vi "MacroFileIO.vi"(0 "New Path IN":path, 1 "MacroFileIO_Command":T3, 5 "Settings File Name IN":string, 7 "Settings Data IN":T2[](array[typedef]), 9 "Setting File Type":T1=enum."Configuration Settings", 11 "Error In":errorcluster, 12 "Macro Text IN":string) -> (3 "File IO Cancelled/NotFound?":bool, 4 "Macro File Path OUT":path, 6 "Temp File path":path, 10 "List of Settings Files in Temp":string[](array[string]), 14 "Macro Text OUT":string, 15 "Error Out":errorcluster)   [LabVIEW 2012]
doc: "SciScan 1.2 160622"
uses:
  MacroFileIO_Commands.ctl
  Custom Controls and Typedefs/GFG Variable for IO.ctl
  Custom Controls/Setting File Types.ctl
  Common Macro VIs/Macro Zip Load_Save_Command.ctl
  INI/settingsIO/Settings IO_Commands.ctl
  GFG/GFGpathGet.vi
  GFG/GFG library.lvlib
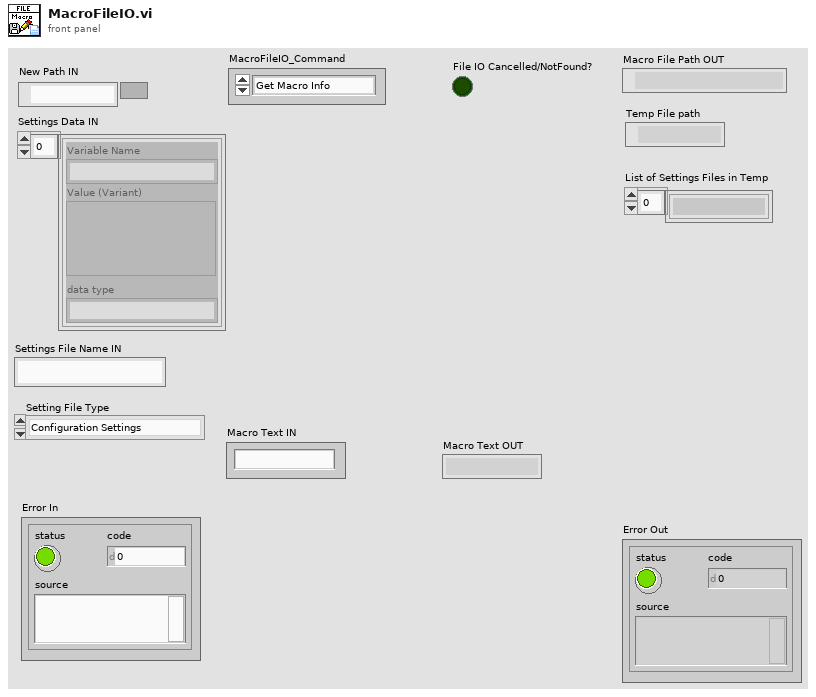
[diagram p1: front panel]
types:
  T1 = typedef "Setting File Types.ctl" = enum16{"2D.Frame.Scan.Settings", "2D.Line.Scan.Settings", "Z.Stack.Settings", "HW Settings", "Configuration Settings", "Unknown Settings", "Fast.Z.Settings"}
  T2 = typedef "GFG Variable for IO.ctl" = cluster{"Variable Name":string, "Value (Variant)":variant, "data type":string}
  T3 = typedef "MacroFileIO_Commands.ctl" = enum16{"Get Macro Info", "Initialize", "New Macro", "Load Macro", "Save", "Save in today's folder", "Update Settings File", "Add Settings File", "Delete Settings File", "Update Macro Text", "Save As", "Read Temp File"}
  T4 = enum16{"open", "replace", "create", "open or create", "replace or create", "replace or create with confirmation"}
  T5 = typedef "Macro Zip Load_Save_Command.ctl" = enum16{"Save zip in recordings folder", "Load macro from zip folder"}
  T6 = typedef "Settings IO_Commands.ctl" = enum16{"Write HW Settings", "Write Config Settings", "Read HW Settings", "Read Config Settings", "Write Line-Scan Settings", "Write Frame-Scan Settings", "Write Z-Stack Settings", "Read Line-Scan Settings", "Read Frame-Scan Settings", "Read Z-Stack Settings", "Read Fast-Z Settings", "Write Fast-Z Settings"}
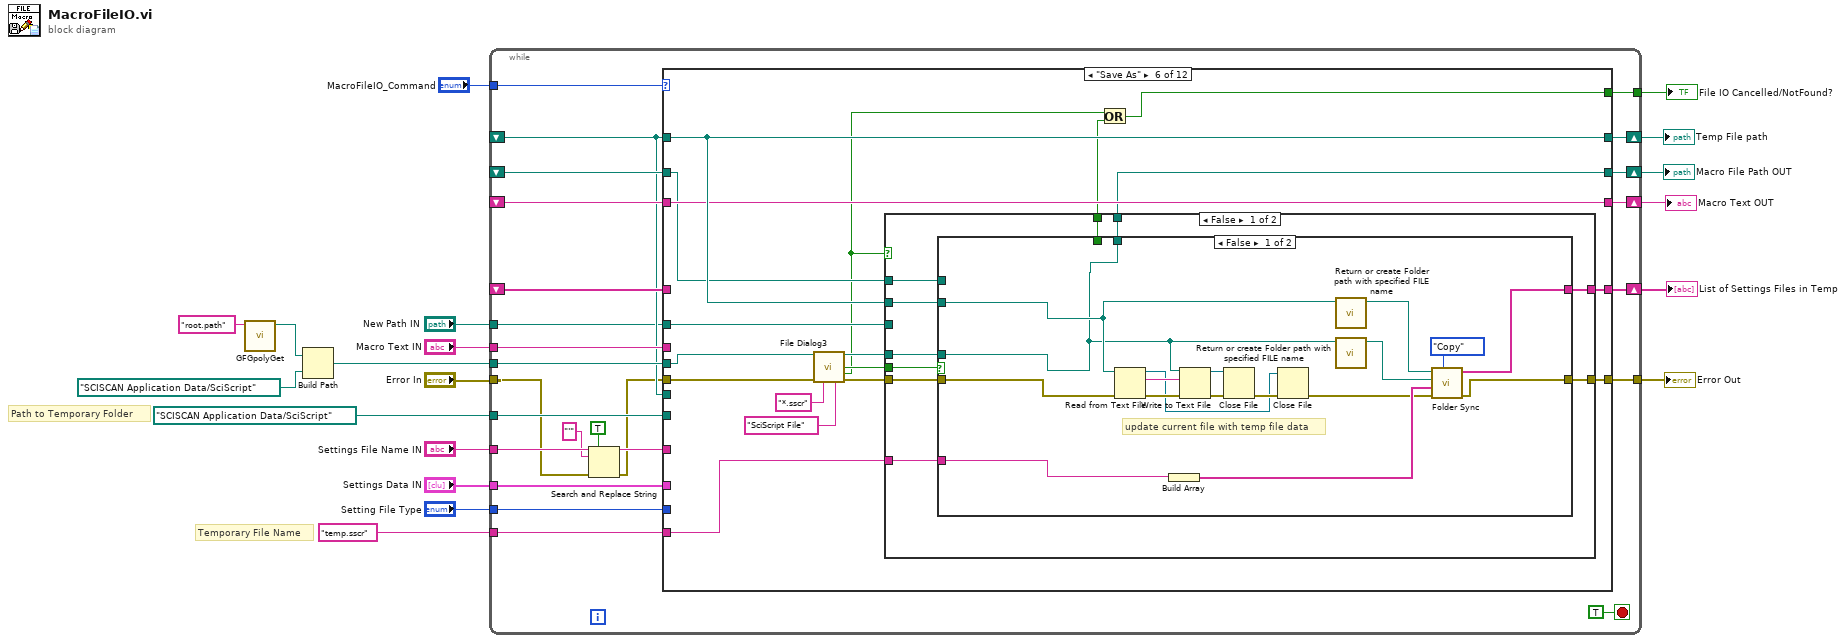
[diagram p0: block diagram]
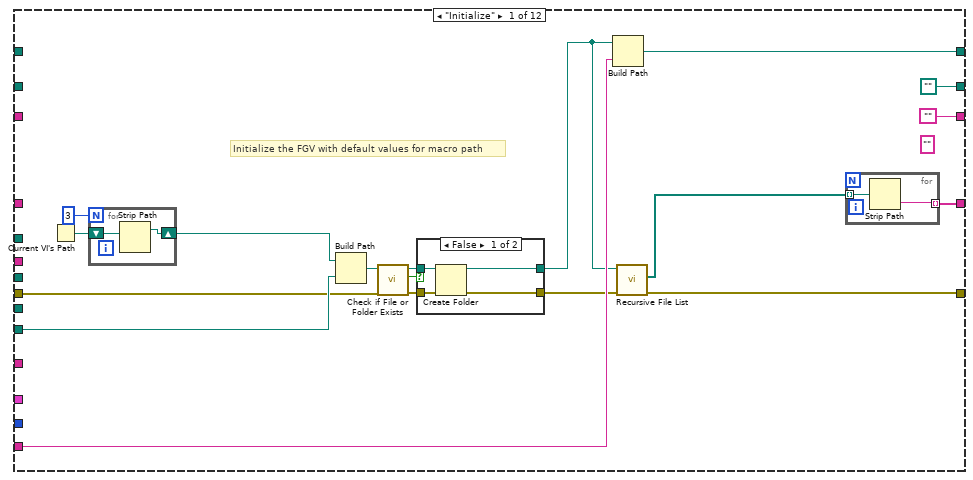
[diagram p2: hidden frame]
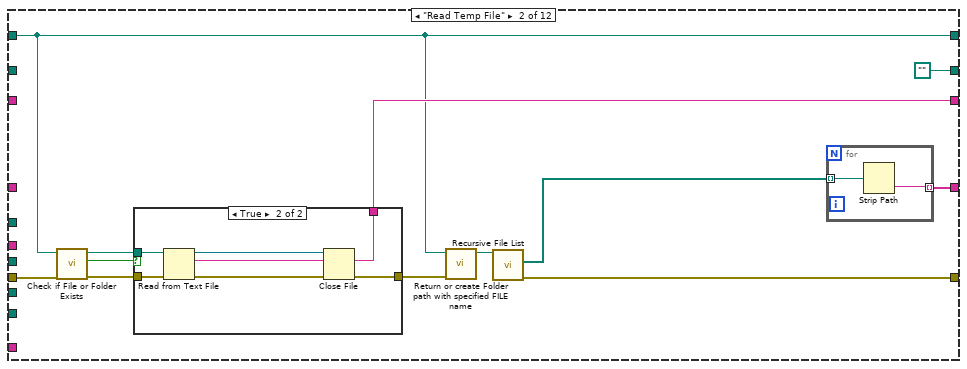
[diagram p4: hidden frame]
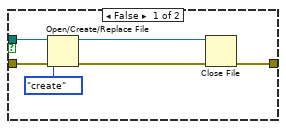
[diagram p5: hidden frame]
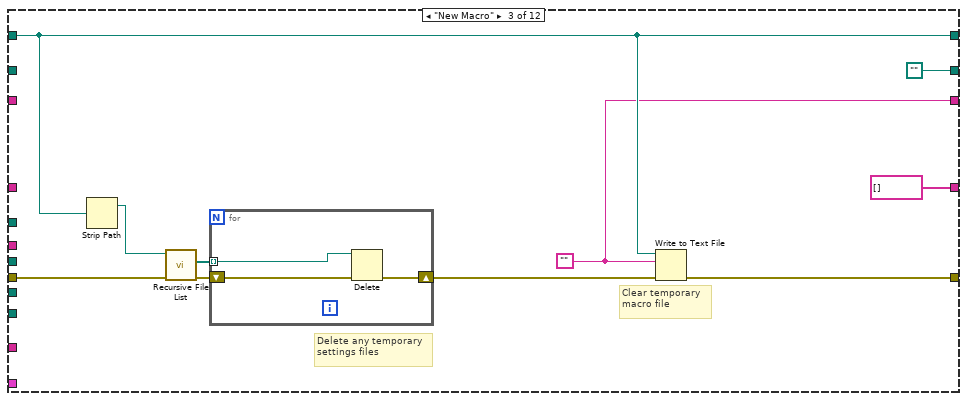
[diagram p6: hidden frame]
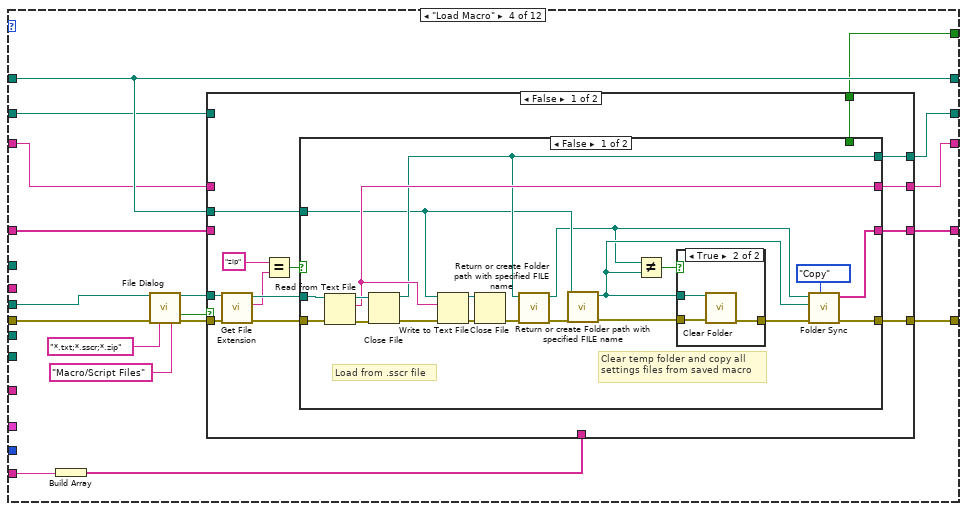
[diagram p7: hidden frame]
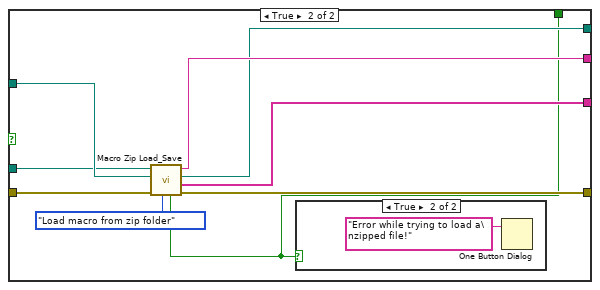
[diagram p9: hidden frame]
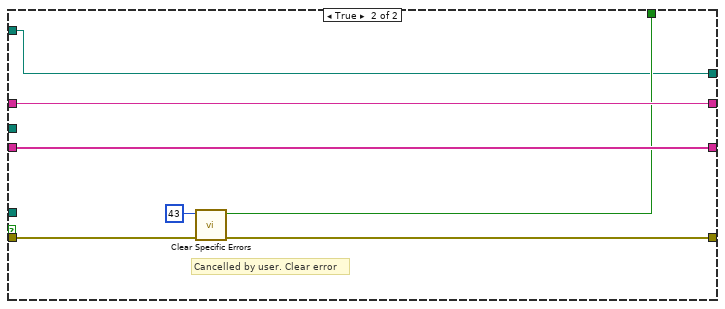
[diagram p11: hidden frame]
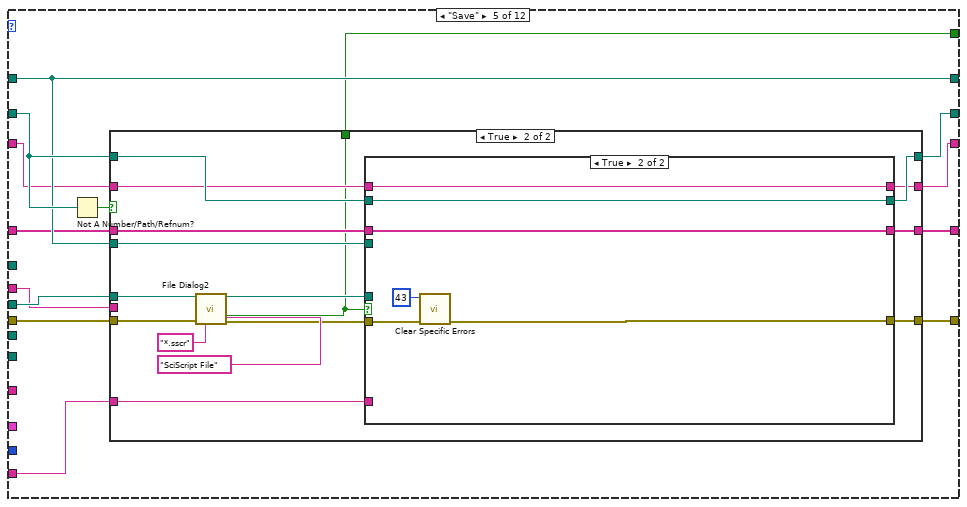
[diagram p12: hidden frame]
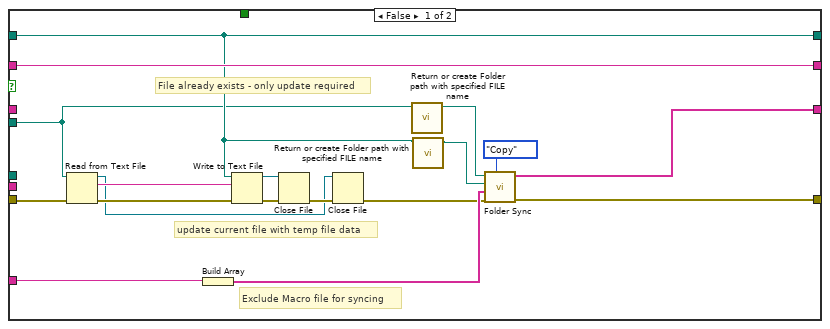
[diagram p13: hidden frame]
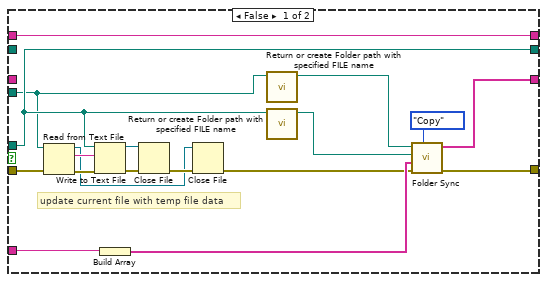
[diagram p14: hidden frame]
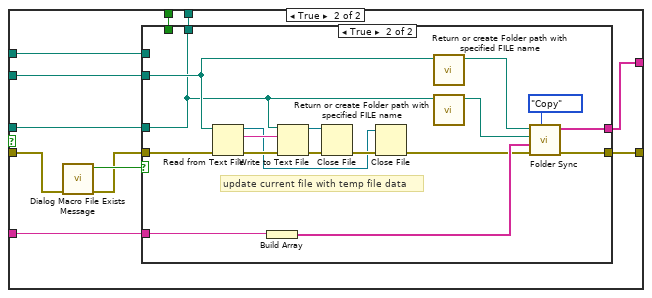
[diagram p15: hidden frame]
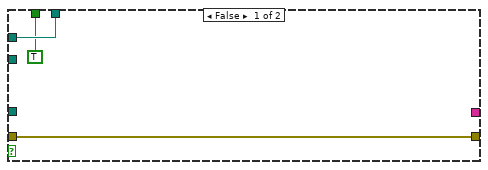
[diagram p16: hidden frame]
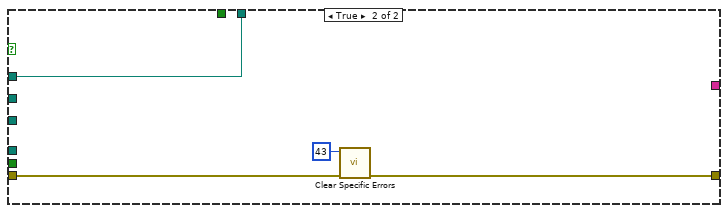
[diagram p17: hidden frame]
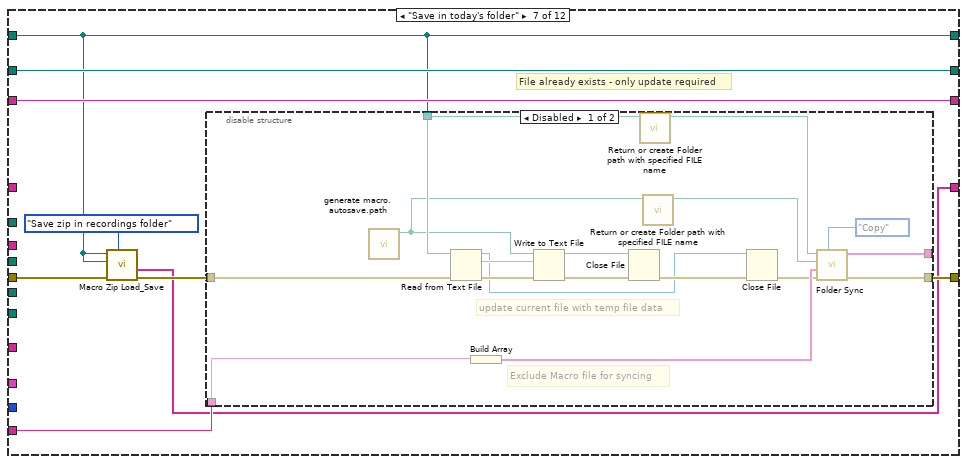
[diagram p18: hidden frame]
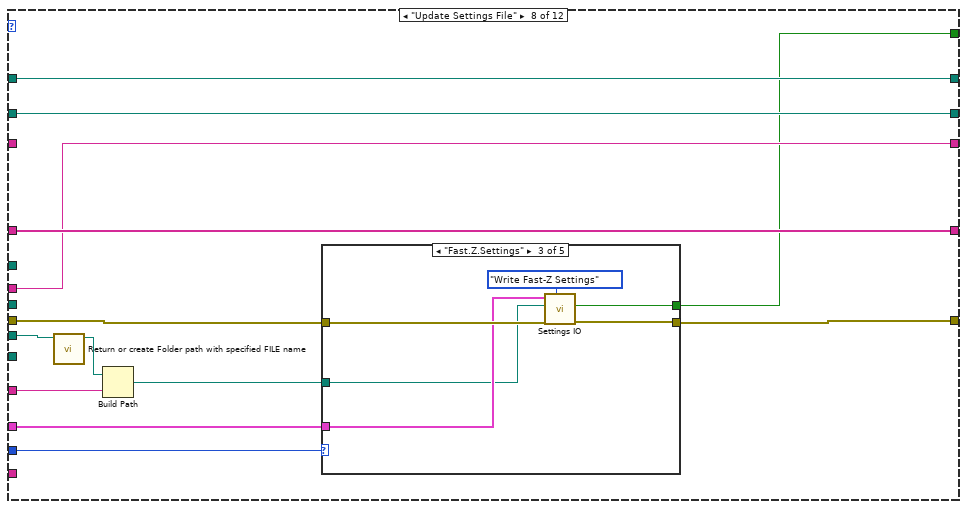
[diagram p20: hidden frame]
diagram:
  # "Temporary File Name"
  # "Path to Temporary Folder"
  n1 = call-poly "GFGpolyGet.vi"("Variable Name in"="root.path") -> ("Path"=w4:path)  [unwired: 8 in, 2 out]
  n2 = Build Path(base path=w4, name or relative path=path "SCISCAN Application Data/SciScript" ("Path IN")) -> (appended path=w3:path)
  n3 = while {
    tunnel: "MacroFileIO_Command" -> [w43]
    tunnel: "Error In" -> [w23]
    tunnel: [w41] -> w18
    tunnel: path "SCISCAN Application Data/SciScript" ("Path IN") -> [w40]
    shift-right: [w39] -> w10
    shift-left: _ -> [w28]
    shift-right: [w38] -> w16
    shift-left: _ -> [w37]
    tunnel: "temp.sscr" ("name or relative path") -> [w36]
    tunnel: "Macro Text IN" -> [w35]
    shift-right: [w34] -> w14
    shift-left: _ -> [w33]
    tunnel: "Settings Data IN" -> [w32]
    tunnel: "Setting File Type" -> [w31]
    shift-right: [w30] -> w9
    shift-left: _ -> [w29]
    tunnel: "Settings File Name IN" -> [w27]
    tunnel: [w21] -> w7
    tunnel: w3 -> [w42]
    tunnel: "New Path IN" -> [w20]
    stop <- TRUE stop-if-true
    n4 = Search and Replace String(replace all?=TRUE ("replace all? (F)"), input string=w27, search string="'", error in=w23) -> (result string=w24:string, error out=w22:errorcluster)  [unwired: 4 in, 2 out]
    n5 = case shown="\"Save As\"" w43 {
      tunnel: w22 -> [w61 w77 w104 w129 w195 w265 w340 w368 w405 w412 w443 w459]
      tunnel: w42 -> [_ _ _ w122 w196 w266 _ _ _ _ _ _]
      tunnel: [w46 w75 w107 w124 w194 w273 w344 w373 w402 w417 w448 w459] -> w41
      tunnel: w40 -> [w62 _ _ _ _ _ _ _ _ _ _ _]
      tunnel: [w48 w74 w106 w121 w190 w272 w337 w370 w403 w414 w449 w461] -> w39
      tunnel: w28 -> [_ w74 w106 w121 w190 w272 w337 w370 w403 w414 w449 w461]
      tunnel: [path "" path "" path "" w123 w193 w260 w343 w375 w407 w419 w452 w460] -> w38
      tunnel: w37 -> [_ _ _ w112 w192 w261 w343 w375 w407 w419 w452 w460]
      tunnel: w36 -> [w60 _ _ w120 w189 w271 w342 _ _ _ _ _]
      tunnel: w35 -> [_ _ _ _ w191 _ _ w371 w404 w415 w450 _]
      tunnel: [w57 w83 string[] [] ("List of Files Copied/Moved") w118 w188 w270 w336 w372 w406 w416 w451 w458] -> w34
      tunnel: w33 -> [_ _ _ w117 w187 _ _ w372 w406 w416 w451 w458]
      tunnel: w32 -> [_ _ _ _ _ _ _ w374 _ w418 _ _]
      tunnel: w31 -> [_ _ _ _ _ _ _ w369 _ w413 _ _]
      tunnel: ["" w79 w99 w116 w186 w269 w341 w371 w404 w415 w450 w457] -> w30
      tunnel: w29 -> [_ _ _ w115 w185 w269 w341 _ _ _ _ w457]
      tunnel: w28 -> [_ _ _ _ _ _ _ w366 _ w411 w446 _]
      tunnel: w24 -> [_ _ _ _ _ _ _ w365 _ w409 w445 _]
      tunnel: [_ _ _ w113 w184 w256 _ w363 _ _ _ _] -> w21
      tunnel: w20 -> [_ _ _ _ _ w268 _ _ _ _ _ _]
      frame "Initialize" {
        (unwired) "" ("Macro Text IN")
        # "Initialize the FGV with default values for macro path"
        n6 = Current VI's Path() -> (path=w52:path)
        n7 = for {
          N: 3 -> [_]
          shift-right: [w63] -> w50
          shift-left: w52 -> [w64]
          n8 = Strip Path(path=w64) -> (stripped path=w63:path)  [unwired: 1 out]
        }
        n9 = Build Path(base path=w50, name or relative path=w62) -> (appended path=w56:path)
        n10 = call <vilib>:"Check if File or Folder Exists.vi"("error in (no error)"=w61, "path"=w56) -> ("error out"=w53:errorcluster, "file or folder exists?"=w55:bool, "dup path"=w54:path)  [unwired: 7 in]
        n11 = case shown="False" w55 {
          tunnel: w54 -> [w67 w69]
          tunnel: w53 -> [w68 w70]
          tunnel: [w65 w70] -> w59
          tunnel: [w66 w69] -> w49
          frame False {
            n12 = Create Folder(path (use dialog)=w67, error in=w68) -> (created path=w66:path, error out=w65:errorcluster)  [unwired: 1 in, 1 out]
          }
          frame True {
          }
        }
        n13 = Build Path(base path=w49, name or relative path=w60) -> (appended path=w48:path)
        n14 = call <vilib>:"Recursive File List.vi"("error in (no error)"=w59, "Folder Path"=w49) -> ("error out"=w46:errorcluster, "All Files in Dir"=w58:path[])  [unwired: 5 in, 3 out]
        n15 = for {
          tunnel: w58 -> [w72] mode=indexing
          tunnel: [w71] -> w57 mode=indexing
          n16 = Strip Path(path=w72) -> (name=w71:string)  [unwired: 1 out]
        }
      }
      frame "Read Temp File" {
        n17 = call <vilib>:"Check if File or Folder Exists.vi"("error in (no error)"=w77, "path"=w74) -> ("error out"=w78:errorcluster, "file or folder exists?"=w81:bool, "dup path"=w80:path)  [unwired: 7 in]
        n18 = case shown="True" w81 {
          tunnel: w80 -> [w90 w96]
          tunnel: [_ w95] -> w79
          tunnel: w78 -> [w89 w92]
          tunnel: [w85 w91] -> w76
          frame False {
            n19 = Open/Create/Replace File(file path (use dialog)=w90, error in=w89, operation (0:open)=T4."create") -> (refnum out=w86:refnum<file>, error out=w87:errorcluster)  [unwired: 3 in, 1 out]
            n20 = Close File(refnum=w86, error in=w87) -> (error out=w85:errorcluster)  [unwired: 1 out]
          }
          frame True {
            n21 = Read from Text File(file (use dialog)=w96, error in=w92) -> (refnum out=w93:refnum<file>, text=w95:string, error out=w94:errorcluster)  [unwired: 2 in, 1 out]
            n22 = Close File(refnum=w93, error in=w94) -> (error out=w91:errorcluster)  [unwired: 1 out]
          }
        }
        n23 = call "Return or create Folder path with specified FILE name.vi"("error in (no error)"=w76, "File Path IN"=w74) -> ("Folder Path OUT"=w82:path)  [unwired: 8 in, 1 out]
        n24 = call <vilib>:"Recursive File List.vi"("Folder Path"=w82) -> ("error out"=w75:errorcluster, "All Files in Dir"=w84:path[])  [unwired: 6 in, 3 out]
        n25 = for {
          tunnel: w84 -> [w98] mode=indexing
          tunnel: [w97] -> w83 mode=indexing
          n26 = Strip Path(path=w98) -> (name=w97:string)  [unwired: 1 out]
        }
      }
      frame "New Macro" {
        w99 = ""
        # "Clear temporary macro file"
        # "Delete any temporary settings files"
        n27 = Strip Path(path=w106) -> (stripped path=w105:path)  [unwired: 1 out]
        n28 = call <vilib>:"Recursive File List.vi"("error in (no error)"=w104, "Folder Path"=w105) -> ("error out"=w103:errorcluster, "All Files in Dir"=w102:path[])  [unwired: 5 in, 3 out]
        n29 = for {
          shift-right: [w109] -> w101
          shift-left: w103 -> [w111]
          tunnel: w102 -> [w110] mode=indexing
          n30 = Delete(path (use dialog)=w110, error in=w111) -> (error out=w109:errorcluster)  [unwired: 3 in, 2 out]
        }
        n31 = Write to Text File(file (use dialog)=w106, text=w99, error in=w101) -> (error out=w107:errorcluster)  [unwired: 1 in, 2 out]
      }
      frame "Load Macro" {
        n32 = Build Array(w120) -> (w119:string[])
        n33 = call "File Dialog"("start path"=w122, "error in"=w129, "pattern (all files)"="*.txt;*.sscr;*.zip", "pattern label"="Macro/Script Files") -> ("selected path"=w126:path, "cancelled"=w114:bool, "error out"=w125:errorcluster)  [unwired: 8 in, 1 out]
        n34 = case shown="False" w114 {
          tunnel: w126 -> [w137 _]
          tunnel: w125 -> [w136 w183]
          tunnel: [w142 w181] -> w124
          tunnel: [w139 w177] -> w123
          tunnel: w121 -> [w138 _]
          tunnel: w119 -> [_ _]
          tunnel: [w141 w180] -> w118
          tunnel: w117 -> [_ w180]
          tunnel: [w140 w179] -> w116
          tunnel: w115 -> [_ w179]
          tunnel: [w130 w178] -> w113
          tunnel: w112 -> [_ w177]
          frame False {
            n35 = call <vilib>:"Get File Extension.vi"("error in (no error)"=w136, "file"=w137) -> ("error out"=w135:errorcluster, "lowercase file extension"=w132:string, "dup file"=w134:path)  [unwired: 6 in, 1 out]
            n36 = Equal?(x="zip" ("lowercase file extension"), y=w132) -> (x = y?=w133:bool)
            n37 = case shown="False" w133 {
              tunnel: w135 -> [w160 w174]
              tunnel: w134 -> [w159 w172]
              tunnel: [w153 w168] -> w142
              tunnel: [w152 w169] -> w141
              tunnel: [w151 w171] -> w140
              tunnel: [w149 w170] -> w139
              tunnel: w138 -> [w147 w173]
              tunnel: [_ w167] -> w130
              frame False {
                # "Load from .sscr file"
                # "Clear temp folder and copy all \nsettings files from saved macro"
                n38 = Read from Text File(file (use dialog)=w159, error in=w160) -> (refnum out=w161:refnum<file>, text=w151:string, error out=w162:errorcluster)  [unwired: 2 in, 1 out]
                n39 = Close File(refnum=w161, error in=w162) -> (path=w149:path, error out=w158:errorcluster)
                n40 = Write to Text File(file (use dialog)=w147, text=w151, error in=w158) -> (refnum out=w156:refnum<file>, error out=w157:errorcluster)  [unwired: 1 in, 1 out]
                n41 = Close File(refnum=w156, error in=w157) -> (error out=w150:errorcluster)  [unwired: 1 out]
                n42 = call "Return or create Folder path with specified FILE name.vi"("error in (no error)"=w150, "File Path IN"=w149) -> ("error out"=w148:errorcluster, "Folder Path OUT"=w144:path)  [unwired: 8 in]
                n43 = call "Return or create Folder path with specified FILE name.vi"("error in (no error)"=w148, "File Path IN"=w147) -> ("error out"=w146:errorcluster, "Folder Path OUT"=w145:path)  [unwired: 8 in]
                n44 = Not Equal?(x=w144, y=w145) -> (x != y?=w143:bool)
                n45 = case shown="True" w143 {
                  tunnel: [w163 w166] -> w154
                  tunnel: w146 -> [w163 w165]
                  tunnel: w145 -> [_ w164]
                  frame False {
                  }
                  frame True {
                    n46 = call "Clear Folder.vi"("error in (no error)"=w165, "Path"=w164) -> ("error out"=w166:errorcluster)  [unwired: 9 in]
                  }
                }
                n47 = call "Folder Sync.vi"("Copy(default)/Move"=enum16{"Copy", "Move"}."Copy", "error in (no error)"=w154, "Destination Folder (To be modified)"=w145, "Source Folder"=w144) -> ("error out"=w153:errorcluster, "List of Files Copied/Moved"=w152:string[])  [unwired: 6 in]
              }
              frame True {
                n48 = call "Macro Zip Load_Save.vi"("Macro Zip Load_Save Command"=Macro_Zip_Load_Save_Command."Load macro from zip folder", "error in (no error)"=w174, "Macro temp file path"=w173, "source file path (*.sscr or *.zip)"=w172) -> ("error out"=w168:errorcluster, "List of Settings Files in Temp"=w169:string[], "Macro File path OUT"=w170:path, "Macro Text Out"=w171:string, "Load Error?"=w167:bool)  [unwired: 3 in]
                n49 = case shown="True" w167 {
                  frame False {
                  }
                  frame True {
                    n50 = One Button Dialog(message="Error while trying to load a\nzipped file!") -> ()  [unwired: 1 in, 1 out]
                  }
                }
              }
            }
          }
          frame True {
            # "Cancelled by user. Clear error"
            n51 = call "Clear Specific Errors.vi"("Error In"=w183, "Error number In"=43) -> ("Error Out"=w181:errorcluster, "Error Cleared?"=w178:bool)  [unwired: 8 in]
          }
        }
      }
      frame "Save" {
        n52 = Not A Number/Path/Refnum?(number/path/refnum=w192) -> (NaN/Path/Refnum?=w197:bool)
        n53 = case shown="True" w197 {
          tunnel: w196 -> [_ w225]
          tunnel: w195 -> [w215 w229]
          tunnel: [w205 w227] -> w194
          tunnel: [w202 w223] -> w193
          tunnel: w192 -> [w202 w224]
          tunnel: w191 -> [_ _]
          tunnel: w190 -> [w201 w219]
          tunnel: w189 -> [w208 w220]
          tunnel: [w204 w222] -> w188
          tunnel: w187 -> [_ w221]
          tunnel: [w203 w218] -> w186
          tunnel: w185 -> [w203 w217]
          tunnel: [_ w216] -> w184
          frame False {
            # "update current file with temp file data"
            # "Exclude Macro file for syncing"
            # "File already exists - only update required"
            n54 = Read from Text File(file (use dialog)=w201, error in=w215) -> (refnum out=w209:refnum<file>, text=w211:string, error out=w212:errorcluster)  [unwired: 2 in, 1 out]
            n55 = Build Array(w208) -> (w207:string[])
            n56 = Write to Text File(file (use dialog)=w202, text=w211, error in=w212) -> (refnum out=w213:refnum<file>, error out=w214:errorcluster)  [unwired: 1 in, 1 out]
            n57 = Close File(refnum=w213, error in=w214) -> (error out=w210:errorcluster)  [unwired: 1 out]
            n58 = Close File(refnum=w209, error in=w210) -> (error out=w200:errorcluster)  [unwired: 1 out]
            n59 = call "Return or create Folder path with specified FILE name.vi"("File Path IN"=w201) -> ("Folder Path OUT"=w198:path)  [unwired: 9 in, 1 out]
            n60 = call "Return or create Folder path with specified FILE name.vi"("File Path IN"=w202) -> ("Folder Path OUT"=w199:path)  [unwired: 9 in, 1 out]
            n61 = call "Folder Sync.vi"("Copy(default)/Move"=enum16{"Copy", "Move"}."Copy", "error in (no error)"=w200, "Exclusion File List"=w207, "Destination Folder (To be modified)"=w199, "Source Folder"=w198) -> ("error out"=w205:errorcluster, "List of Files Copied/Moved"=w204:string[])  [unwired: 5 in]
          }
          frame True {
            n62 = call "File Dialog2"("start path"=w225, "error in"=w229, "pattern (all files)"="*.sscr", "pattern label"="SciScript File") -> ("selected path"=w226:path, "cancelled"=w216:bool, "error out"=w228:errorcluster)  [unwired: 8 in, 1 out]
            n63 = case shown="True" w216 {
              tunnel: w228 -> [w242 w254]
              tunnel: [w241 w253] -> w227
              tunnel: w226 -> [w236 _]
              tunnel: w224 -> [_ w252]
              tunnel: [w236 w252] -> w223
              tunnel: [w240 w251] -> w222
              tunnel: w221 -> [_ w251]
              tunnel: w220 -> [w239 _]
              tunnel: w219 -> [w235 _]
              tunnel: [w237 w250] -> w218
              tunnel: w217 -> [w237 w250]
              frame False {
                # "update current file with temp file data"
                n64 = Read from Text File(file (use dialog)=w235, error in=w242) -> (refnum out=w244:refnum<file>, text=w246:string, error out=w247:errorcluster)  [unwired: 2 in, 1 out]
                n65 = Write to Text File(file (use dialog)=w236, text=w246, error in=w247) -> (refnum out=w248:refnum<file>, error out=w249:errorcluster)  [unwired: 1 in, 1 out]
                n66 = Build Array(w239) -> (w238:string[])
                n67 = Close File(refnum=w248, error in=w249) -> (error out=w245:errorcluster)  [unwired: 1 out]
                n68 = Close File(refnum=w244, error in=w245) -> (error out=w232:errorcluster)  [unwired: 1 out]
                n69 = call "Return or create Folder path with specified FILE name.vi"("File Path IN"=w235) -> ("Folder Path OUT"=w233:path)  [unwired: 9 in, 1 out]
                n70 = call "Return or create Folder path with specified FILE name.vi"("File Path IN"=w236) -> ("Folder Path OUT"=w234:path)  [unwired: 9 in, 1 out]
                n71 = call "Folder Sync.vi"("Copy(default)/Move"=enum16{"Copy", "Move"}."Copy", "error in (no error)"=w232, "Exclusion File List"=w238, "Destination Folder (To be modified)"=w234, "Source Folder"=w233) -> ("error out"=w241:errorcluster, "List of Files Copied/Moved"=w240:string[])  [unwired: 5 in]
              }
              frame True {
                n72 = call "Clear Specific Errors.vi"("Error In"=w254, "Error number In"=43) -> ("Error Out"=w253:errorcluster)  [unwired: 8 in, 1 out]
              }
            }
          }
        }
      }
      frame "Save As" {
        n73 = call "File Dialog3"("start path"=w266, "error in"=w265, "pattern (all files)"="*.sscr", "pattern label"="SciScript File") -> ("selected path"=w263:path, "exists"=w259:bool, "cancelled"=w258:bool, "error out"=w264:errorcluster)  [unwired: 8 in]
        n74 = case shown="False" w258 {
          tunnel: [w283 w332] -> w273
          tunnel: w272 -> [w282 _]
          tunnel: w271 -> [w281 _]
          tunnel: [w280 _] -> w270
          tunnel: w268 -> [_ _]
          tunnel: w264 -> [w275 w334]
          tunnel: w263 -> [w279 _]
          tunnel: w261 -> [w277 w333]
          tunnel: [w278 w333] -> w260
          tunnel: w259 -> [w276 _]
          tunnel: [w274 _] -> w257
          frame False {
            n75 = case shown="False" w276 {
              tunnel: [w285 w311] -> w283
              tunnel: w282 -> [w300 w310]
              tunnel: w281 -> [w298 w309]
              tunnel: [w284 w308] -> w280
              tunnel: w275 -> [w299 w302]
              tunnel: w279 -> [w297 w307]
              tunnel: [w297 w305] -> w278
              tunnel: w277 -> [_ w306]
              tunnel: [_ w304] -> w274
              frame False {
                # "update current file with temp file data"
                n76 = Read from Text File(file (use dialog)=w300, error in=w299) -> (refnum out=w291:refnum<file>, text=w293:string, error out=w294:errorcluster)  [unwired: 2 in, 1 out]
                n77 = Build Array(w298) -> (w289:string[])
                n78 = Write to Text File(file (use dialog)=w297, text=w293, error in=w294) -> (refnum out=w295:refnum<file>, error out=w296:errorcluster)  [unwired: 1 in, 1 out]
                n79 = Close File(refnum=w295, error in=w296) -> (error out=w292:errorcluster)  [unwired: 1 out]
                n80 = Close File(refnum=w291, error in=w292) -> (error out=w286:errorcluster)  [unwired: 1 out]
                n81 = call "Return or create Folder path with specified FILE name.vi"("File Path IN"=w300) -> ("Folder Path OUT"=w287:path)  [unwired: 9 in, 1 out]
                n82 = call "Return or create Folder path with specified FILE name.vi"("File Path IN"=w297) -> ("Folder Path OUT"=w288:path)  [unwired: 9 in, 1 out]
                n83 = call "Folder Sync.vi"("Copy(default)/Move"=enum16{"Copy", "Move"}."Copy", "error in (no error)"=w286, "Exclusion File List"=w289, "Destination Folder (To be modified)"=w288, "Source Folder"=w287) -> ("error out"=w285:errorcluster, "List of Files Copied/Moved"=w284:string[])  [unwired: 5 in]
              }
              frame True {
                n84 = call "Dialog Macro File Exists Message.vi"("error in (no error)"=w302) -> ("error out"=w301:errorcluster, "Confirmed?"=w303:bool)  [unwired: 9 in]
                n85 = case shown="True" w303 {
                  tunnel: [w313 w331] -> w311
                  tunnel: w310 -> [_ w316]
                  tunnel: w309 -> [_ w330]
                  tunnel: [_ w329] -> w308
                  tunnel: w301 -> [w313 w317]
                  tunnel: w307 -> [_ w315]
                  tunnel: w306 -> [w314 _]
                  tunnel: [w314 w315] -> w305
                  tunnel: [TRUE _] -> w304
                  frame False {
                  }
                  frame True {
                    # "update current file with temp file data"
                    n86 = Read from Text File(file (use dialog)=w316, error in=w317) -> (refnum out=w323:refnum<file>, text=w325:string, error out=w326:errorcluster)  [unwired: 2 in, 1 out]
                    n87 = Build Array(w330) -> (w321:string[])
                    n88 = Write to Text File(file (use dialog)=w315, text=w325, error in=w326) -> (refnum out=w327:refnum<file>, error out=w328:errorcluster)  [unwired: 1 in, 1 out]
                    n89 = Close File(refnum=w327, error in=w328) -> (error out=w324:errorcluster)  [unwired: 1 out]
                    n90 = Close File(refnum=w323, error in=w324) -> (error out=w318:errorcluster)  [unwired: 1 out]
                    n91 = call "Return or create Folder path with specified FILE name.vi"("File Path IN"=w316) -> ("Folder Path OUT"=w319:path)  [unwired: 9 in, 1 out]
                    n92 = call "Return or create Folder path with specified FILE name.vi"("File Path IN"=w315) -> ("Folder Path OUT"=w320:path)  [unwired: 9 in, 1 out]
                    n93 = call "Folder Sync.vi"("Copy(default)/Move"=enum16{"Copy", "Move"}."Copy", "error in (no error)"=w318, "Exclusion File List"=w321, "Destination Folder (To be modified)"=w320, "Source Folder"=w319) -> ("error out"=w331:errorcluster, "List of Files Copied/Moved"=w329:string[])  [unwired: 5 in]
                  }
                }
              }
            }
          }
          frame True {
            n94 = call "Clear Specific Errors.vi"("Error In"=w334, "Error number In"=43) -> ("Error Out"=w332:errorcluster)  [unwired: 8 in, 1 out]
          }
        }
        n95 = Or(x=w258, y=w257) -> (x .or. y?=w256:bool)
      }
      frame "Save in today's folder" {
        # "File already exists - only update required"
        n96 = call "Macro Zip Load_Save.vi"("Macro Zip Load_Save Command"=Macro_Zip_Load_Save_Command."Save zip in recordings folder", "error in (no error)"=w340, "Macro temp file path"=w337, "source file path (*.sscr or *.zip)"=w337) -> ("error out"=w339:errorcluster, "List of Settings Files in Temp"=w336:string[])  [unwired: 3 in, 3 out]
        n97 = disable-structure shown="Disabled" {
          disable-tunnel: w339 -> [w361 w362]
          disable-tunnel: [w360 w362] -> w344
          disable-tunnel: w337 -> [w359 _]
          disable-tunnel: w342 -> [w358 _]
          disable-tunnel: [w357 _] -> _
          frame Disabled {
            # "update current file with temp file data"
            # "Exclude Macro file for syncing"
            n98 = call "generate macro.autosave.path.vi"() -> ("macro.autosave.path"=w346:path)  [unwired: 10 in, 1 out]
            n99 = Read from Text File(file (use dialog)=w359, error in=w361) -> (refnum out=w351:refnum<file>, text=w353:string, error out=w354:errorcluster)  [unwired: 2 in, 1 out]
            n100 = Build Array(w358) -> (w350:string[])
            n101 = Write to Text File(file (use dialog)=w346, text=w353, error in=w354) -> (refnum out=w355:refnum<file>, error out=w356:errorcluster)  [unwired: 1 in, 1 out]
            n102 = Close File(refnum=w355, error in=w356) -> (error out=w352:errorcluster)  [unwired: 1 out]
            n103 = call "Return or create Folder path with specified FILE name.vi"("File Path IN"=w359) -> ("Folder Path OUT"=w347:path)  [unwired: 9 in, 1 out]
            n104 = call "Return or create Folder path with specified FILE name.vi"("File Path IN"=w346) -> ("Folder Path OUT"=w345:path)  [unwired: 9 in, 1 out]
            n105 = Close File(refnum=w351, error in=w352) -> (error out=w348:errorcluster)  [unwired: 1 out]
            n106 = call "Folder Sync.vi"("Copy(default)/Move"=enum16{"Copy", "Move"}."Copy", "error in (no error)"=w348, "Exclusion File List"=w350, "Destination Folder (To be modified)"=w345, "Source Folder"=w347) -> ("error out"=w360:errorcluster, "List of Files Copied/Moved"=w357:string[])  [unwired: 5 in]
          }
          frame Enabled {
          }
        }
      }
      frame "Update Settings File" {
        n107 = call "Return or create Folder path with specified FILE name.vi"("File Path IN"=w366) -> ("Folder Path OUT"=w367:path)  [unwired: 9 in, 1 out]
        n108 = Build Path(base path=w367, name or relative path=w365) -> (appended path=w364:path)
        n109 = case shown="\"Fast.Z.Settings\"" w369 {
          tunnel: w368 -> [w380 w386 w393 w395 w400]
          tunnel: w374 -> [w379 w385 w392 _ w399]
          tunnel: [w377 w383 w390 w395 w398] -> w373
          tunnel: w364 -> [w378 w384 w391 _ w397]
          tunnel: [w376 w382 w389 TRUE ("Cancelled/Not Found?") w396] -> w363
          frame "2D.Frame.Scan.Settings" {
            n110 = call "Settings IO.vi"("SettingsFileIO_Commands"=Settings_IO_Commands."Write Frame-Scan Settings", "Error In"=w380, "File Path (for scan specific settings)"=w378, "Settings Array IN"=w379) -> ("Error Out"=w377:errorcluster, "Cancelled?"=w376:bool)  [unwired: 5 in, 1 out]
          }
          frame "Z.Stack.Settings" {
            n111 = call "Settings IO.vi"("SettingsFileIO_Commands"=Settings_IO_Commands."Write Z-Stack Settings", "Error In"=w386, "File Path (for scan specific settings)"=w384, "Settings Array IN"=w385) -> ("Error Out"=w383:errorcluster, "Cancelled?"=w382:bool)  [unwired: 5 in, 1 out]
          }
          frame "Fast.Z.Settings" {
            n112 = call "Settings IO.vi"("SettingsFileIO_Commands"=Settings_IO_Commands."Write Fast-Z Settings", "Error In"=w393, "File Path (for scan specific settings)"=w391, "Settings Array IN"=w392) -> ("Error Out"=w390:errorcluster, "Cancelled?"=w389:bool)  [unwired: 5 in, 1 out]
          }
          frame Default {
          }
          frame "2D.Line.Scan.Settings" {
            n113 = call "Settings IO.vi"("SettingsFileIO_Commands"=Settings_IO_Commands."Write Line-Scan Settings", "Error In"=w400, "File Path (for scan specific settings)"=w397, "Settings Array IN"=w399) -> ("Error Out"=w398:errorcluster, "Cancelled?"=w396:bool)  [unwired: 5 in, 1 out]
          }
        }
      }
      frame "Update Macro Text" {
        # "Write macro text\nfile"
        n114 = Write to Text File(file (use dialog)=w403, text=w404, error in=w405) -> (error out=w402:errorcluster)  [unwired: 1 in, 2 out]
      }
      frame "Add Settings File" {
        n115 = call "Return or create Folder path with specified FILE name.vi"("File Path IN"=w411) -> ("Folder Path OUT"=w410:path)  [unwired: 9 in, 1 out]
        n116 = Build Path(base path=w410, name or relative path=w409) -> (appended path=w408:path)
        n117 = case shown="\"Fast.Z.Settings\"" w413 {
          tunnel: w412 -> [w423 w428 w433 w435 w439]
          tunnel: w418 -> [w422 w427 w432 _ w438]
          tunnel: [w420 w426 w431 w435 w437] -> w417
          tunnel: w408 -> [w421 w425 w430 _ w436]
          frame "2D.Frame.Scan.Settings" {
            n118 = call "Settings IO.vi"("SettingsFileIO_Commands"=Settings_IO_Commands."Write Frame-Scan Settings", "Error In"=w423, "File Path (for scan specific settings)"=w421, "Settings Array IN"=w422) -> ("Error Out"=w420:errorcluster)  [unwired: 5 in, 2 out]
          }
          frame "Z.Stack.Settings" {
            n119 = call "Settings IO.vi"("SettingsFileIO_Commands"=Settings_IO_Commands."Write Z-Stack Settings", "Error In"=w428, "File Path (for scan specific settings)"=w425, "Settings Array IN"=w427) -> ("Error Out"=w426:errorcluster)  [unwired: 5 in, 2 out]
          }
          frame "Fast.Z.Settings" {
            n120 = call "Settings IO.vi"("SettingsFileIO_Commands"=Settings_IO_Commands."Write Fast-Z Settings", "Error In"=w433, "File Path (for scan specific settings)"=w430, "Settings Array IN"=w432) -> ("Error Out"=w431:errorcluster)  [unwired: 5 in, 2 out]
          }
          frame Default {
          }
          frame "2D.Line.Scan.Settings" {
            n121 = call "Settings IO.vi"("SettingsFileIO_Commands"=Settings_IO_Commands."Write Line-Scan Settings", "Error In"=w439, "File Path (for scan specific settings)"=w436, "Settings Array IN"=w438) -> ("Error Out"=w437:errorcluster)  [unwired: 5 in, 2 out]
          }
        }
      }
      frame "Delete Settings File" {
        n122 = call "Return or create Folder path with specified FILE name.vi"("File Path IN"=w446) -> ("Folder Path OUT"=w447:path)  [unwired: 9 in, 1 out]
        n123 = Build Path(base path=w447, name or relative path=w445) -> (appended path=w442:path)
        n124 = call <vilib>:"Check if File or Folder Exists.vi"("error in (no error)"=w443, "path"=w442) -> ("error out"=w444:errorcluster, "file or folder exists?"=w441:bool)  [unwired: 7 in, 1 out]
        n125 = case shown="False" w441 {
          tunnel: w444 -> [w453 w456]
          tunnel: [w453 w455] -> w448
          tunnel: w442 -> [_ w454]
          frame False {
            # "FIle not found!\nDo nothing"
          }
          frame True {
            n126 = Delete(path (use dialog)=w454, error in=w456) -> (error out=w455:errorcluster)  [unwired: 3 in, 2 out]
          }
        }
      }
      frame "Get Macro Info", Default {
      }
    }
  }
  "Error Out" <- w18
  "Macro File Path OUT" <- w16
  "List of Settings Files in Temp" <- w14
  "Temp File path" <- w10
  "Macro Text OUT" <- w9
  "File IO Cancelled/NotFound?" <- w7
